vi "test_curr_new.vi"() -> ()   [LabVIEW 2015]
panel:
  in  "Stop Button":bool
  out "Current value (A)":string
  in  "Open Database":bool
  out "Waveform Chart":dbl(graph)
  in  "Refresh":bool
  in  "Acquisition frequency (s)":enum32{"600", "60", "10", "1"}(ring)=enum."1"
  in  "Close VI":bool
  in  "Run Test":bool
  out "error out":errorcluster[](array[cluster])
  in  "Measure time (s)":string="300"
  # "Insert measure parameters and then click \"Run test\""
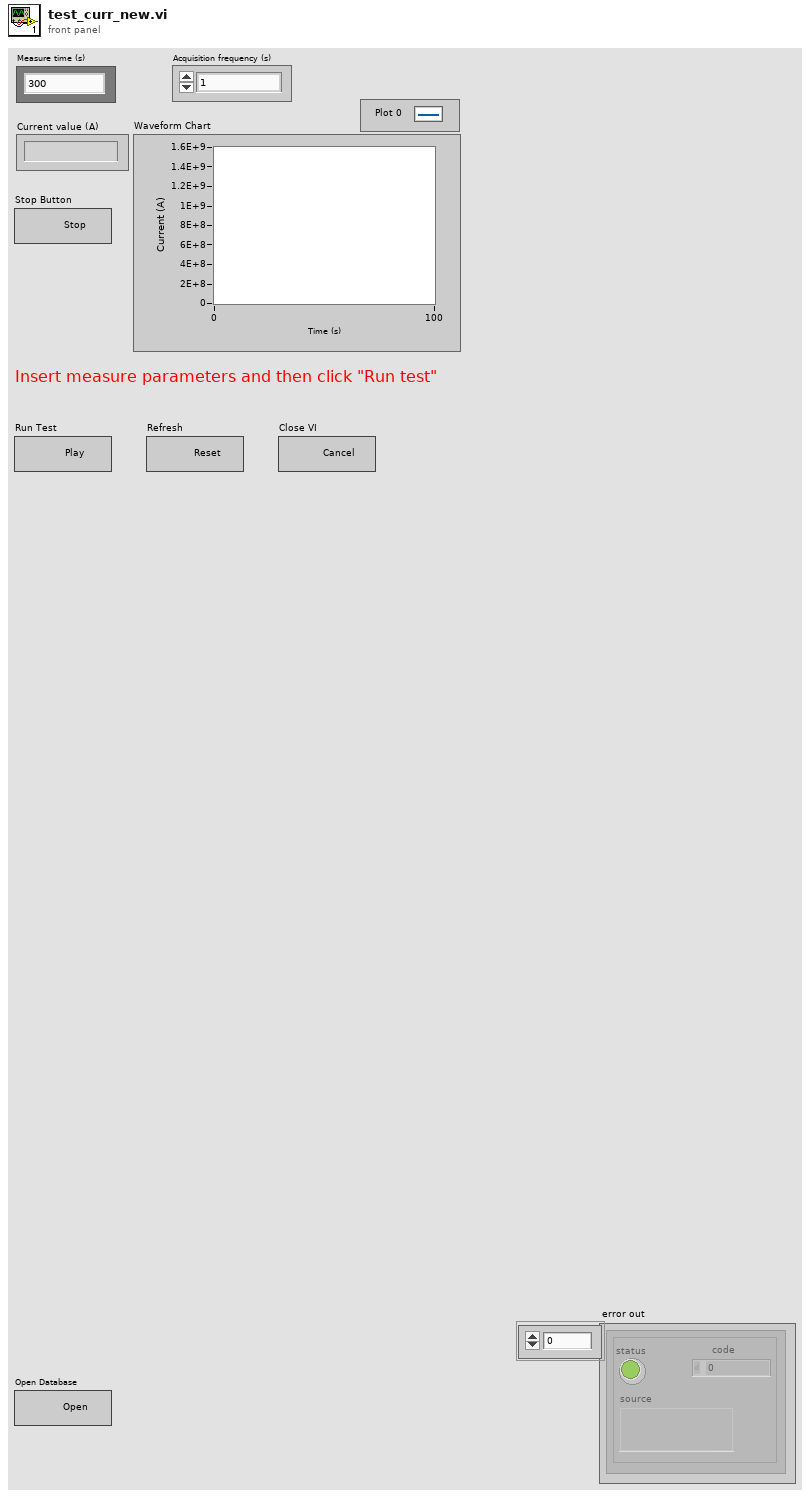
[diagram p1: front panel]
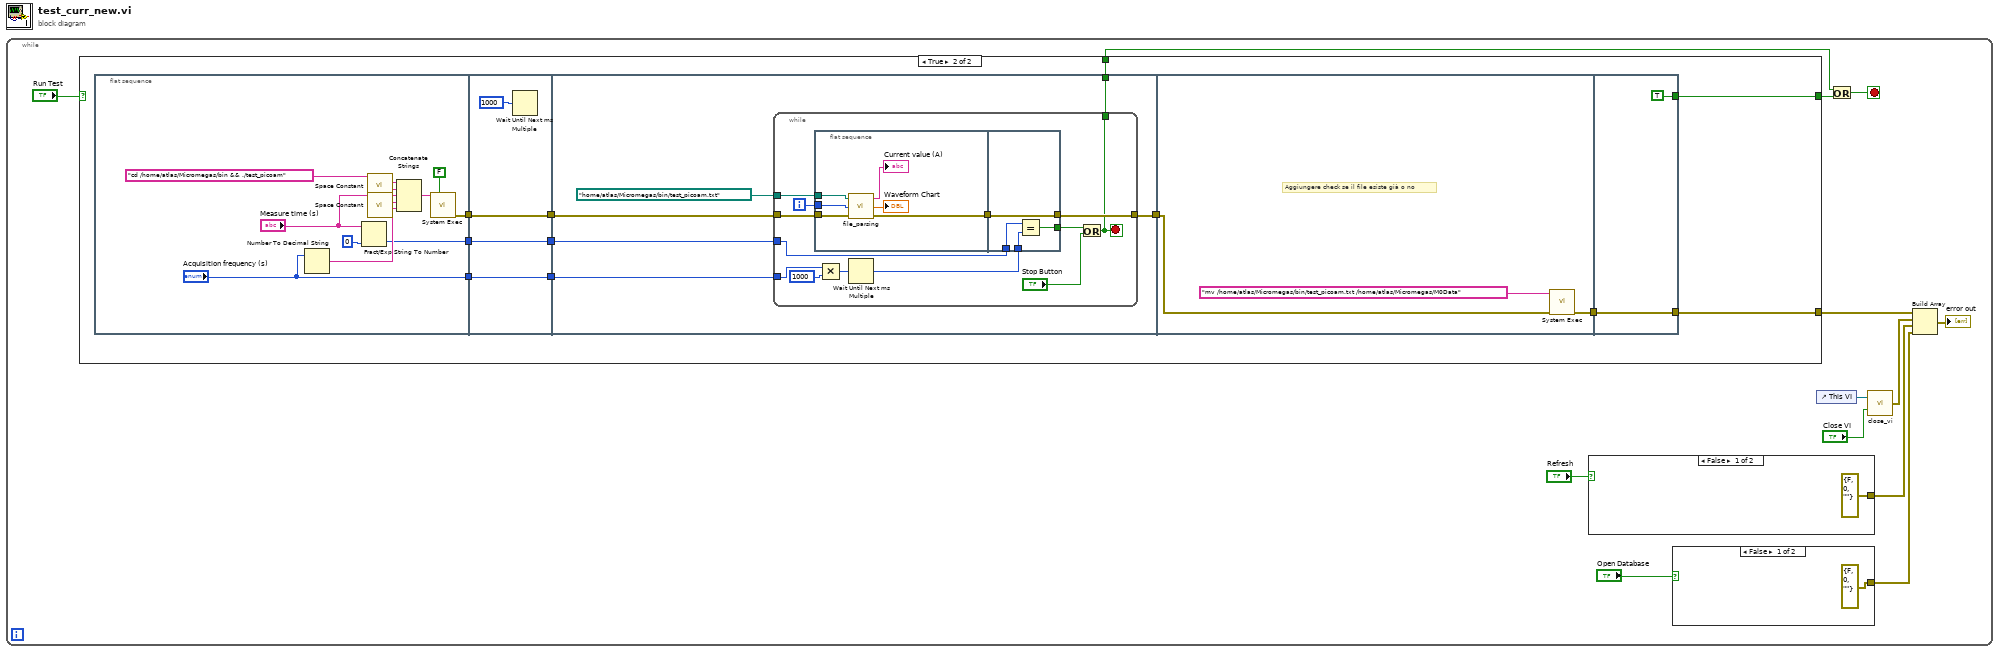
[diagram p0: block diagram]
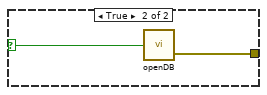
[diagram p2: hidden frame]
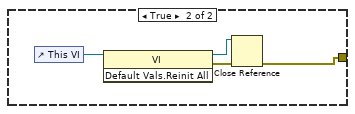
[diagram p3: hidden frame]
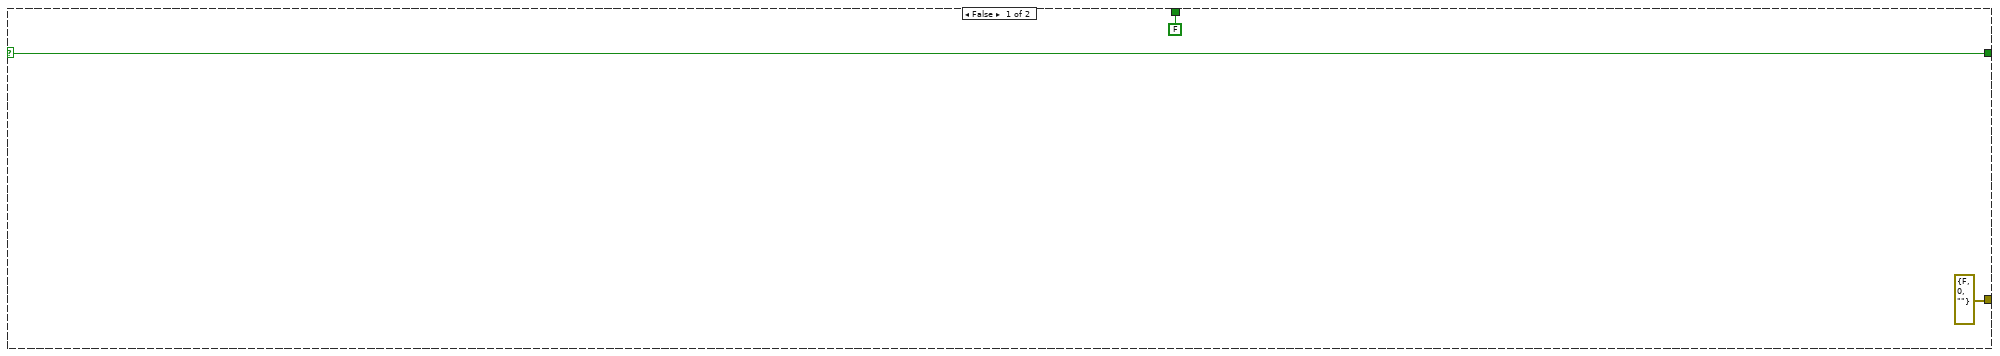
[diagram p4: hidden frame]
diagram:
  n1 = while {
    stop <- w1 stop-if-true
    n2 = case shown="True" "Run Test" {
      selector: "Run Test" -> [w24 _]
      tunnel: [w24 w35] -> w3
      tunnel: [errorcluster {"status"=FALSE, "code"=0, "source"=""} ("error out") w32] -> w11
      tunnel: [FALSE w25] -> w2
      frame False {
      }
      frame True {
        n3 = flat-sequence {
          tunnel: [w46] -> w31
          tunnel: ["Acquisition frequency (s)"] -> w29
          tunnel: [w37] -> w27
          tunnel: w31 -> [w50]
          tunnel: [w50] -> w34
          tunnel: [w48] -> w30
          tunnel: w29 -> [w48]
          tunnel: [w47] -> w28
          tunnel: w27 -> [w47]
          tunnel: w34 -> [w55]
          tunnel: w30 -> [w54]
          tunnel: w28 -> [w53]
          tunnel: [w52] -> w26
          tunnel: [w51] -> w25
          tunnel: [w81] -> w33
          tunnel: w26 -> [w80]
          tunnel: [TRUE] -> w35
          tunnel: [w83] -> w32
          tunnel: w33 -> [w83]
          frame #0 {
            n4 = Number To Decimal String(number="Acquisition frequency (s)") -> (decimal integer string=w45:string)  [unwired: 1 in]
            n5 = Fract/Exp String To Number(string="Measure time (s)", default (0 dbl)=0) -> (number=w37:i32)  [unwired: 2 in, 1 out]
            n6 = call <vilib>:"Space Constant.vi"() -> ("String"=w43:string)
            n7 = call <vilib>:"Space Constant.vi"() -> ("String"=w44:string)
            n8 = Concatenate Strings("cd /home/atlas/Micromegas/bin && ./test_picoam" ("String"), w43, "Measure time (s)", w44, w45) -> (w41:string)
            n9 = call <vilib>:"System Exec.vi"("wait until completion? (T)"=FALSE, "command line"=w41) -> ("error out"=w46:errorcluster)  [unwired: 6 in, 3 out]
          }
          frame #1 {
            n10 = Wait Until Next ms Multiple(millisecond multiple=u32 1000) -> ()  [unwired: 1 out]
          }
          frame #2 {
            n11 = while {
              tunnel: path "/home/atlas/Micromegas/bin/test_picoam.txt" -> [w64]
              tunnel: w55 -> [w65]
              tunnel: w54 -> [w67]
              tunnel: w53 -> [w62]
              tunnel: [w61] -> w52
              tunnel: [w57] -> w51
              i -> [w66]
              stop <- w57 stop-if-true
              n12 = flat-sequence {
                tunnel: w66 -> [w75]
                tunnel: w65 -> [w74]
                tunnel: w64 -> [w73]
                tunnel: [w70] -> w60
                tunnel: w63 -> [w77]
                tunnel: w62 -> [w76]
                tunnel: [w79] -> w58
                tunnel: [w78] -> w61
                tunnel: w60 -> [w78]
                frame #0 {
                  n13 = call "file_parsing.vi"("error in"=w74, "line index"=w75, "File Path Control"=w73) -> ("error out"=w70:errorcluster, "Waveform Chart"=→"Waveform Chart":dbl, "String"=→"Current value (A)":string)
                }
                frame #1 {
                  n14 = Equal?(x=w76, y=w77) -> (x = y?=w79:bool)
                }
              }
              n15 = Multiply(x=w67, y=1000) -> (x*y=w68:u32)
              n16 = Wait Until Next ms Multiple(millisecond multiple=w68) -> (millisecond timer value=w63:u32)
              n17 = Or(x=w58, y="Stop Button") -> (x .or. y?=w57:bool)
            }
          }
          frame #3 {
            # "Aggiungere check se il file esiste già o no"
            n18 = call <vilib>:"System Exec.vi"("error in (no error)"=w80, "command line"="mv /home/atlas/Micromegas/bin/test_picoam.txt /home/atlas/Micromegas/M0Data") -> ("error out"=w81:errorcluster)  [unwired: 6 in, 3 out]
          }
          frame #4 {
          }
        }
      }
    }
    n19 = case shown="False" "Refresh" {
      tunnel: [errorcluster {"status"=FALSE, "code"=0, "source"=""} ("error out") w18] -> w10
      frame False {
      }
      frame True {
        n20 = control-ref of="This VI"() -> (w21:refnum<vi>)
        n21 = invoke class="VI" method="Default Vals.Reinit All"(reference=w21) -> (reference out=w20:refnum<vi>, error out=w19:errorcluster)  [unwired: 2 in, 1 out]
        n22 = Close Reference(reference=w20, error in (no error)=w19) -> (error out=w18:errorcluster)
      }
    }
    n23 = case shown="False" "Open Database" {
      selector: "Open Database" -> [_ w16]
      tunnel: [errorcluster {"status"=FALSE, "code"=0, "source"=""} ("error out") w15] -> w7
      frame False {
      }
      frame True {
        n24 = call "openDB.vi"("Open Button"=w16) -> ("error out"=w15:errorcluster)  [unwired: 1 out]
      }
    }
    n25 = control-ref of="This VI"() -> (w6:refnum<vi>)
    n26 = Or(x=w2, y=w3) -> (x .or. y?=w1:bool)
    n27 = call "close_vi.vi"("Process Stop Button"="Close VI", "reference"=w6) -> ("error out"=w4:errorcluster)
    n28 = Build Array(w11, w4, w10, w7) -> (→"error out":errorcluster[])
  }
